vi "Ctor.vi"(7 "Tree":refnum<class "PathTree.lvclass">, 8 "error in (no error)":errorcluster, 10 "Parent":refnum<class "PathTreeNode.lvclass">, 11 "Token":string) -> (0 "error out":errorcluster, 3 "PathTreeNode out":refnum<class "PathTreeNode.lvclass">)   [LabVIEW 2020, in "PathTree.lvlib" / "PathTreeNode.lvclass"]
uses:
  PathTreeNode.lvclass
  PathTree/PathTree.lvclass
  Ref Data.ctl
  PathTreeNode.lvclass/PathTreeNode.ctl
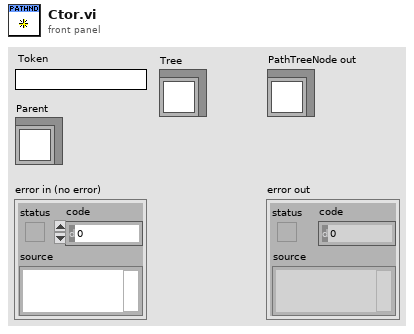
[diagram p1: front panel]
types:
  T1 = typedef "PathTree.lvlib/PathTreeNode.lvclass/Ref Data.ctl" = cluster{"Tree":refnum<class>, "Parent":refnum<class>, "Token":string, "Child Tokens":string[], "Child Nodes":refnum<class>[], "Value":refnum<class>, "Has Value":bool}
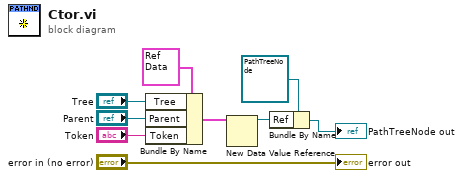
[diagram p0: block diagram]
diagram:
  n1 = Bundle By Name(cluster=T1 {"Tree"=refnum, "Parent"=refnum, "Token"="", "Child Tokens"=[], "Child Nodes"=[], "Value"=refnum, "Has Value"=FALSE} ("Ref Data"), "Tree"="Tree", "Parent"="Parent", "Token"="Token") -> (w3:T1)
  n2 = New Data Value Reference(data value=w3) -> (data value reference=w1:refnum<data-value>)  [unwired: 1 in, 1 out]
  n3 = Bundle By Name(cluster=refnum<class "PathTreeNode.lvclass"> refnum ("PathTreeNode in"), "Ref"=w1) -> (→"PathTreeNode out":refnum<class "PathTreeNode.lvclass">)
  "error out" <- "error in (no error)"
